vi "LED.vi"() -> ()   [LabVIEW 2020]
panel:
  in  "Wait_Constant":dbl
  in  "Color_Start":u32(colorbox)=16776002
  in  "Color Array":u32[](array[colorbox])
  in  "fade constant":dbl
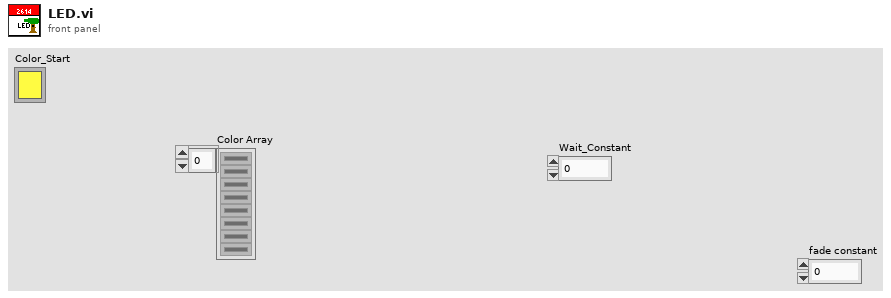
[diagram p1: front panel]
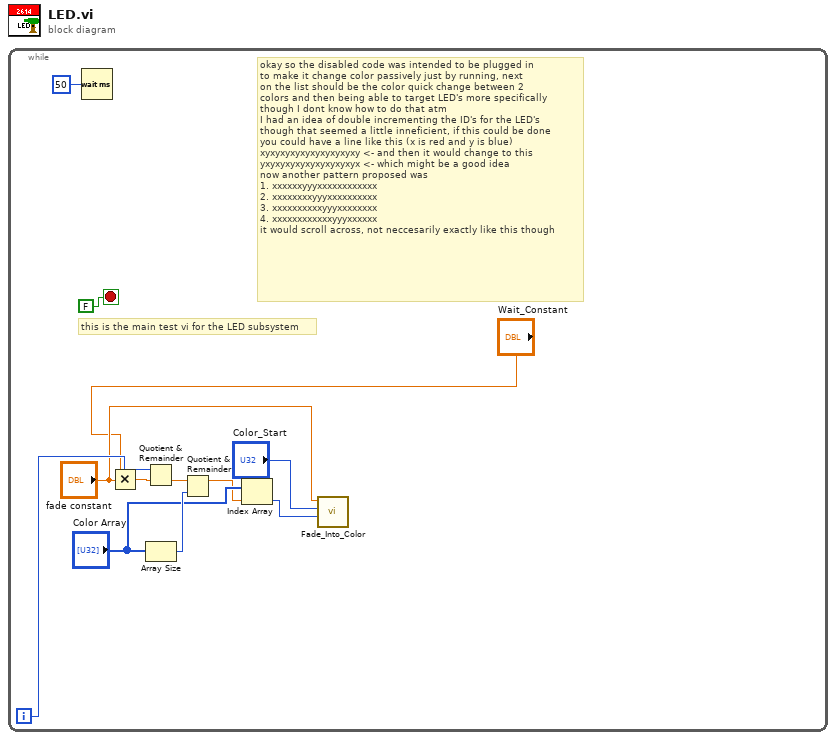
[diagram p0: block diagram]
diagram:
  n1 = while {
    i -> [w10]
    stop <- FALSE stop-if-true
    # "okay so the disabled code was intended to be plugged in\nto make it change color passively just by running, next \non the list should be the color quick change between 2\ncolors and then being able to target LED's more specifically\nthough I dont know how to do that atm\nI had an idea of double incrementing the ID's for the LED's \nthough that seemed a little inneficient, if this could be done \nyou could have a line like this (x is red and y is blue)\nxyxyxyxyxyxyxyxyxyxy <- and then it would change to this\nyxyxyxyxyxyxyxyxyxyx <- which might be a good idea\nnow another pattern proposed was\n1. xxxxxxyyyxxxxxxxxxxxx\n2. xxxxxxxxyyyxxxxxxxxxx\n3. xxxxxxxxxxyyyxxxxxxxx\n4. xxxxxxxxxxxxyyyxxxxxx\nit would scroll across, not neccesarily exactly like this though"
    # "this is the main test vi for the LED subsystem"
    n2 = Wait (ms)(milliseconds to wait=u32 50) -> ()  [unwired: 1 out]
    n3 = Multiply(x="fade constant", y="Wait_Constant") -> (x*y=w3:dbl)
    n4 = Quotient & Remainder(x=w10, y=w3) -> (floor(x/y)=w9:dbl)  [unwired: 1 out]
    n5 = Array Size(array="Color Array") -> (size(s)=w8:i32)
    n6 = Quotient & Remainder(x=w9, y=w8) -> (x-y*floor(x/y)=w6:dbl)  [unwired: 1 out]
    n7 = Index Array(array="Color Array", index=w6) -> (element=w5:u32)
    n8 = call "Fade_Into_Color.vi"("Color_Goal"=w5, "Color_Start"="Color_Start", "fade constant"="fade constant") -> ()  [unwired: 9 in]
  }
